vi "Send.vi"(5 "Record Topic Name?":bool, 7 "Message Priority":T1, 8 "error in (no error)":errorcluster, 9 "Timeout":i32, 10 "Message":refnum<class "Message Interface.lvclass">, 11 "Message Transport Interface in":refnum<class "Message Transport Interface.lvclass">) -> (0 "error out":errorcluster, 2 "Timed Out?":bool, 3 "Message Transport Interface out":refnum<class "Message Transport Interface.lvclass">)   [LabVIEW 2016, in "Stream Mediator.lvlib" / "Message Transport Interface.lvclass"]
doc: "--\nCopyright © 2017 Composed SystemsI All rights reserved.\n\nAuthor: Jon McBee <jon.mcbee@composed.io>\n\nThis library is provided \"AS IS\" ,WITHOUT WARRANTIES OR\nCONDITIONS OF ANY KIND, either express or implied.\n\nComposed Systems -- composed.io\n\nStream 0.0.1.1\nJon McBee - Composed Systems\nCopyright (c) 2017, Composed Systems"
uses:
  <userlib>/Composed Systems/Stream/Mediator/Classes/Message Transport Interface/Message Transport Interface.lvclass
  <userlib>/Composed Systems/Stream/Mediator/Classes/Message Interface/Message Interface.lvclass
  <userlib>/Composed Systems/Stream/Mediator/Classes/Message Transport Interface/Message Priority.ctl
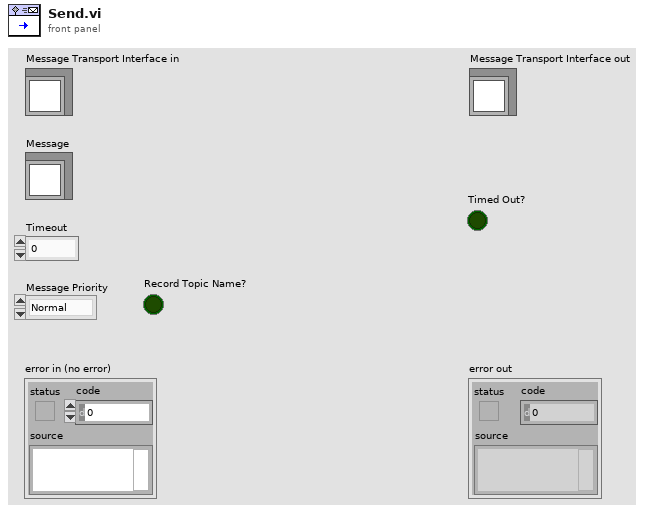
[diagram p1: front panel]
types:
  T1 = typedef "Stream Mediator.lvlib/Message Transport Interface.lvclass/Message Priority.ctl" = enum16{"Normal", "High"}
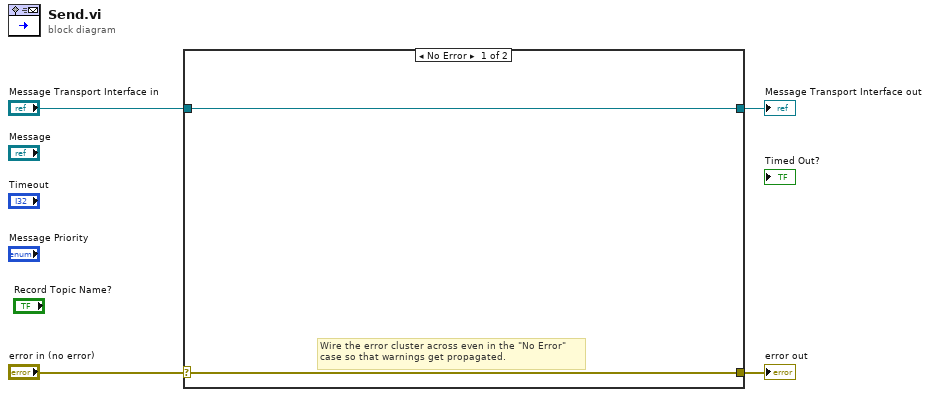
[diagram p0: block diagram]
diagram:
  n1 = case shown="No Error" "error in (no error)" {
    selector: "error in (no error)" -> [w5 w8]
    tunnel: [w5 w8] -> w3
    tunnel: [w6 w7] -> w1
    tunnel: "Message Transport Interface in" -> [w6 w7]
    frame No Error {
      # "Wire the error cluster across even in the \"No Error\"\ncase so that warnings get propagated."
    }
    frame Error {
    }
  }
  "error out" <- w3
  "Message Transport Interface out" <- w1
